vi "Synx2Meas.vi"(8 "error in (no error)":errorcluster, 11 "RingdownPlugin in":refnum<class "EraPlugin.lvclass">) -> (0 "error out":errorcluster, 2 "Measurements":waveform(dbl)[](array[waveform]), 3 "RingdownPlugin out":refnum<class "EraPlugin.lvclass">)   [LabVIEW 2017, in "AppPlugins.lvlib" / "ERAPlugin.lvclass"]
uses:
  EraPlugin.lvclass
  C:/dev/Work/PARTF/Modules/AppPlugins/AppPluginBaseClass/AppPluginsBase.lvclass
  AppPluginBaseClass/AppPluginsBase.lvclass/AppPluginsBase.ctl
  EraPlugin.lvclass/EraPlugin.ctl
  AppPluginBaseClass/Accessors/Read clEvtReportArray.vi
  Accessors/Read RingdownConfig.vi
  <vilib>/Analysis/NI_AALPro.lvlib
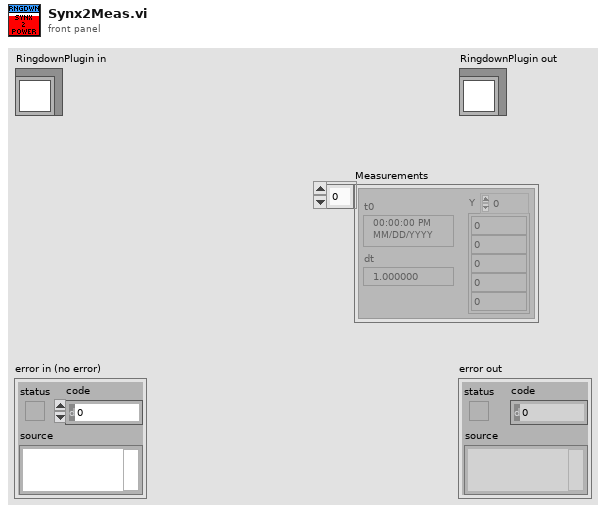
[diagram p1: front panel]
types:
  T1 = typedef "EventPlugins.lvlib/EventPluginBaseClass.lvclass/clEvtReportArray.ctl" = T2[]
  T2 = typedef "EventPlugins.lvlib/EventPluginBaseClass.lvclass/clEvtReport.ctl" = cluster{"Timestamp":dbl, "Synx":cdb[], "Freq":dbl, "ROCOF":dbl, "ID":i16}
  T3 = typedef "AppPlugins.lvlib/ERAPlugin.lvclass/RingdownConfig.ctl" = cluster{"Config":cluster{"p_SysOdr":i32, "dThres":dbl, "Preproc":cluster{"order":i32, "f_lo":dbl, "f_hi":dbl, "R_down":i32}}, "V index":i32, "I index":i32, "PosSeq":bool}
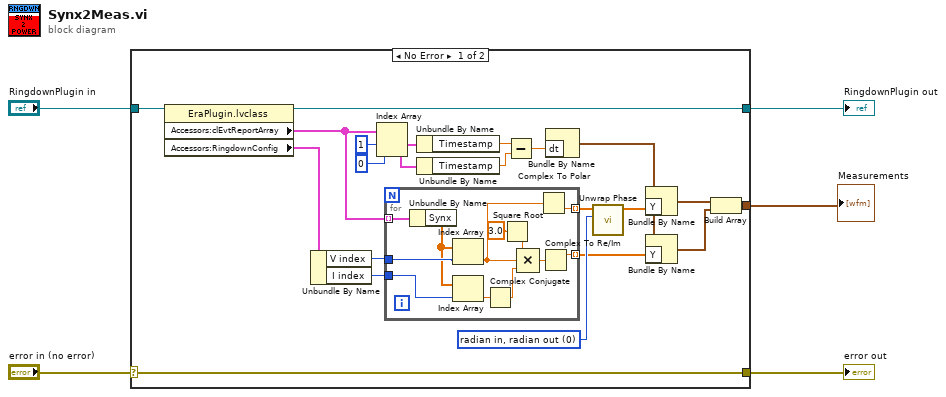
[diagram p0: block diagram]
diagram:
  n1 = case shown="No Error" "error in (no error)" {
    selector: "error in (no error)" -> [w26 w41]
    tunnel: [w26 w41] -> w4
    tunnel: [w25 w40] -> w2
    tunnel: "RingdownPlugin in" -> [w27 w40]
    tunnel: [w6 _] -> w1
    frame No Error {
      w20 = 0 items=["radian in, radian out", "radian in, degree out", "degree in, degree out", "degree in, radian out"] ("phase unit")
      n2 = property class="EraPlugin.lvclass"(reference=w27) -> (reference out=w25:refnum<class "EraPlugin.lvclass">, "Accessors:clEvtReportArray"=w19:T1, "Accessors:RingdownConfig"=w22:T3)  [unwired: 1 in, 1 out]
      n3 = Unbundle By Name(w22) -> ("V index"=w23:i32, "I index"=w24:i32)
      n4 = Index Array(array=w19, index #1=1 ("index"), index #2=0 ("index")) -> (element #1=w16:T2, element #2=w15:T2)
      n5 = for {
        tunnel: w24 -> [w37]
        tunnel: w23 -> [w38]
        tunnel: w19 -> [w39] mode=indexing
        tunnel: [w30] -> w8 mode=indexing
        tunnel: [w28] -> w21 mode=indexing
        n6 = Unbundle By Name(w39) -> ("Synx"=w36:cdb[])
        n7 = Index Array(array=w36, index=w38) -> (element=w29:cdb)
        n8 = Index Array(array=w36, index=w37) -> (element=w35:cdb)
        n9 = Complex Conjugate(1:w35) -> (0:w34:cdb)
        n10 = Square Root(x=3.0) -> (sqrt(x)=w32:dbl)
        n11 = Compound Arithmetic op=MULTIPLY(w32, w29, w34) -> (w33:cdb)
        n12 = Complex To Polar(r * e^(i*theta)=w29) -> (theta=w28:dbl)  [unwired: 1 out]
        n13 = Complex To Re/Im(x + iy=w33) -> (x=w30:dbl)  [unwired: 1 out]
      }
      n14 = Unbundle By Name(w16) -> ("Timestamp"=w14:dbl)
      n15 = Unbundle By Name(w15) -> ("Timestamp"=w13:dbl)
      n16 = Subtract(x=w14, y=w13) -> (x-y=w12:dbl)
      n17 = Bundle By Name("dt"=w12) -> (w10:waveform(dbl))  [unwired: 1 in]
      n18 = call <vilib>:"Unwrap Phase.vi"("phase unit"=w20, "Phase"=w21) -> ("Unwrapped Phase"=w11:dbl[])  [unwired: 8 in, 1 out]
      n19 = Bundle By Name(cluster=w10, "Y"=w11) -> (w9:waveform(dbl))
      n20 = Bundle By Name(cluster=w10, "Y"=w8) -> (w7:waveform(dbl))
      n21 = Build Array(w9, w7) -> (w6:waveform(dbl)[])
    }
    frame Error {
    }
  }
  "error out" <- w4
  "RingdownPlugin out" <- w2
  "Measurements" <- w1
